vi "Computer_Control_Layer.vi"() -> ()   [LabVIEW 2014]
panel:
  out "Queued Array":dbl[][](array[numeric])
  in  "Angles":dbl[](array[numeric])=[0.0, 0.0, 0.0, 0.0, 0.0]
  in  "stop":bool
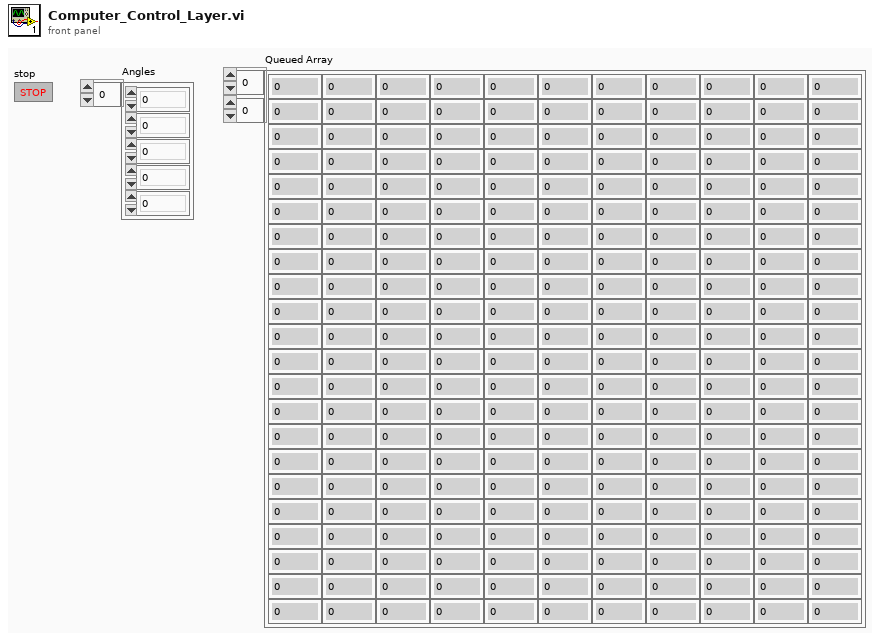
[diagram p1: front panel]
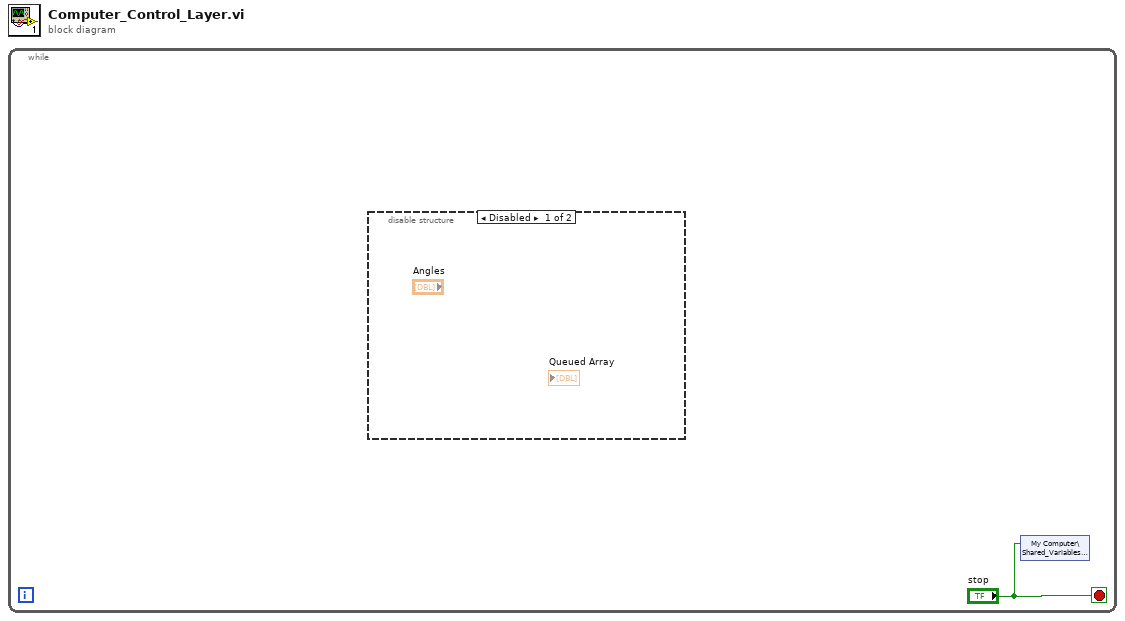
[diagram p0: block diagram]
diagram:
  n1 = while {
    stop <- "stop" stop-if-true
    n2 = disable-structure shown="Disabled" {
      frame Disabled {
      }
      frame Enabled {
      }
    }
    n3 = shared-variable "My Computer\\Shared_Variables.lvlib\\Stop"("stop") -> ()  [unwired: 1 in, 1 out]
  }
